vi "DiffIO Write.vi"(8 "FIFO Indexes.Write":cluster{"Diff I/O Setup":T1[]}, 9 "Command Enabled":bool, 11 "Device Inputs":dbl[](array[numeric])) -> (3 "Diff IO Setup":T2[](array[typedef]) {"Skip Fire Index" max=7; "Angles"."Duration [s]" format="%#_3p"; "Frequency [Hz]" format="%#_3p"})   [LabVIEW 2016, in "DCM Engine.lvlib"]
uses:
  DCM Engine.lvlib
  Built/DCM Classes Packed/Pharlap/C/DCM-Classes.lvlibp/DCM/Diff IO/RT/Setup.ctl
  Built/DCM Classes Packed/Pharlap/C/DCM-Classes.lvlibp/1abvi3w/vi.lib/Powertrain Controls/Device Drivers/DCM/Diff IO/FPGA/Mode.ctl
  Built/DCM Classes Packed/Pharlap/C/DCM-Classes.lvlibp/DCM/Diff IO/RT/Angle Control.ctl
  Shared/Types/DiffIO Setup Indexes.ctl
  Built/DCM Classes Packed/Pharlap/C/DCM-Classes.lvlibp/1abvi3w/vi.lib/Powertrain Controls/Device Drivers/DCM/Diff IO/FPGA/DCM - FPGA - Diff IO.lvlib
  Built/DCM Classes Packed/Pharlap/C/DCM-Classes.lvlibp/DCM/Diff IO/RT/DCM - RT - Diff IO.lvlib
  DCM Shared.lvlib
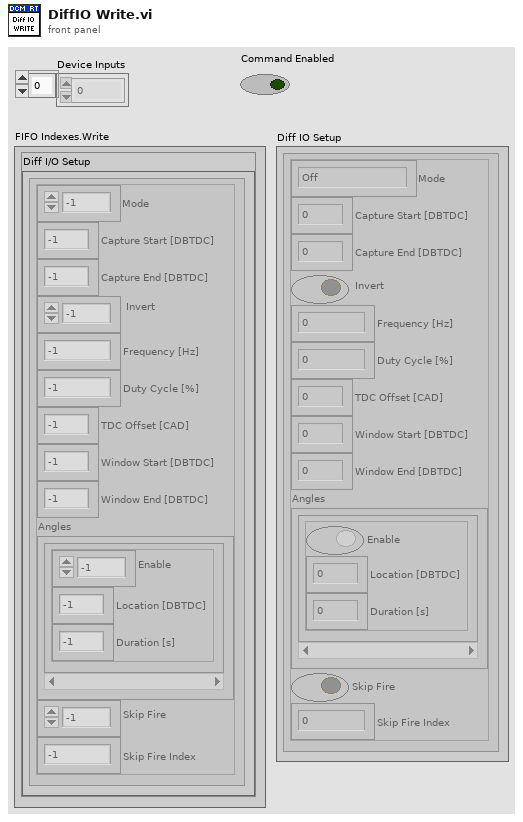
[diagram p1: front panel]
types:
  T1 = typedef "DCM Shared.lvlib/DiffIO Setup Indexes.ctl" = cluster{"Mode":i32, "Capture Start [DBTDC]":i32, "Capture End [DBTDC]":i32, "Invert":i32, "Frequency [Hz]":i32, "Duty Cycle [%]":i32, "TDC Offset [CAD]":i32, "Window Start [DBTDC]":i32, "Window End [DBTDC]":i32, "Angles":cluster{"Enable":i32, "Location [DBTDC]":i32, "Duration [s]":i32}[], "Skip Fire":i32, "Skip Fire Index":i32}
  T2 = typedef "DCM-Classes.lvlibp/DCM - RT - Diff IO.lvlib/Setup.ctl" = cluster{"Mode":T3, "Capture Start [DBTDC]":sgl, "Capture End [DBTDC]":sgl, "Invert":bool, "Frequency [Hz]":sgl, "Duty Cycle [%]":sgl, "TDC Offset [CAD]":sgl, "Window Start [DBTDC]":sgl, "Window End [DBTDC]":sgl, "Angles":T4[], "Skip Fire":bool, "Skip Fire Index":u8}
  T3 = typedef "DCM-Classes.lvlibp/DCM - FPGA - Diff IO.lvlib/Mode.ctl" = enum8{"Off", "Input", "Pulse Width Modulation", "Engine Position Tracking", "Serial Out 1", "Serial Out 2", "EPTx Sync"}
  T4 = typedef "DCM-Classes.lvlibp/DCM - RT - Diff IO.lvlib/Angle Control.ctl" = cluster{"Enable":bool, "Location [DBTDC]":sgl, "Duration [s]":sgl}
  T5 = cluster{"Enable":i32, "Location [DBTDC]":i32, "Duration [s]":i32}[]
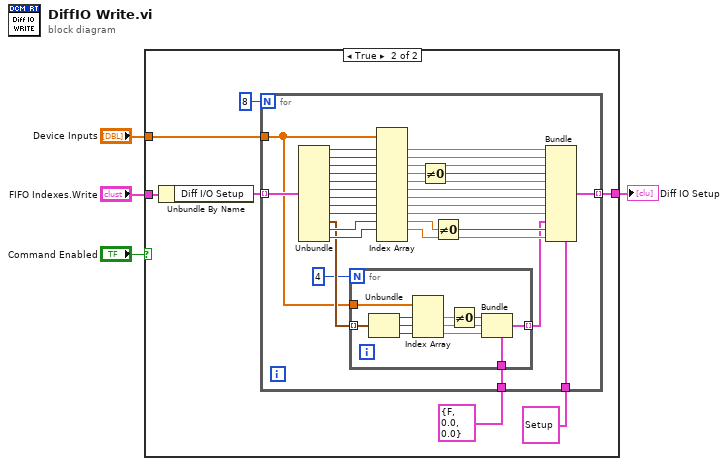
[diagram p0: block diagram]
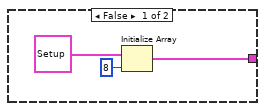
[diagram p2: hidden frame]
diagram:
  n1 = case shown="True" "Command Enabled" {
    tunnel: "Device Inputs" -> [_ w14]
    tunnel: [w5 w12] -> w3
    tunnel: "FIFO Indexes.Write" -> [_ w9]
    frame False {
      n2 = Initialize Array(T2 {"Mode"=enum."Off", "Capture Start [DBTDC]"=0.0, "Capture End [DBTDC]"=0.0, "Invert"=FALSE, "Frequency [Hz]"=0.0, "Duty Cycle [%]"=0.0, "TDC Offset [CAD]"=0.0, "Window Start [DBTDC]"=0.0, "Window End [DBTDC]"=0.0, "Angles"=[{"Enable"=FALSE, "Location [DBTDC]"=0.0, "Duration [s]"=0.0}, {"Enable"=FALSE, "Location [DBTDC]"=0.0, "Duration [s]"=0.0}, {"Enable"=FALSE, "Location [DBTDC]"=0.0, "Duration [s]"=0.0}, {"Enable"=FALSE, "Location [DBTDC]"=0.0, "Duration [s]"=0.0}], "Skip Fire"=FALSE, "Skip Fire Index"=0} ("PWM Control 2"), 8 ("dimension size")) -> (w5:T2[])
    }
    frame True {
      n3 = Unbundle By Name(w9) -> ("Diff I/O Setup"=w13:T1[])
      n4 = for {
        N: 8 -> [_]
        tunnel: w14 -> [w33]
        tunnel: w13 -> [w46] mode=indexing
        tunnel: [w32] -> w12 mode=indexing
        tunnel: T4 {"Enable"=FALSE, "Location [DBTDC]"=0.0, "Duration [s]"=0.0} ("Injection Control") -> [w31]
        tunnel: T2 {"Mode"=enum."Off", "Capture Start [DBTDC]"=0.0, "Capture End [DBTDC]"=0.0, "Invert"=FALSE, "Frequency [Hz]"=0.0, "Duty Cycle [%]"=0.0, "TDC Offset [CAD]"=0.0, "Window Start [DBTDC]"=0.0, "Window End [DBTDC]"=0.0, "Angles"=[{"Enable"=FALSE, "Location [DBTDC]"=0.0, "Duration [s]"=0.0}, {"Enable"=FALSE, "Location [DBTDC]"=0.0, "Duration [s]"=0.0}, {"Enable"=FALSE, "Location [DBTDC]"=0.0, "Duration [s]"=0.0}, {"Enable"=FALSE, "Location [DBTDC]"=0.0, "Duration [s]"=0.0}], "Skip Fire"=FALSE, "Skip Fire Index"=0} ("PWM Control 2") -> [w15]
        n5 = Unbundle(w46) -> ("Mode"=w45:i32, "Capture Start [DBTDC]"=w44:i32, "Capture End [DBTDC]"=w43:i32, "Invert"=w42:i32, "Frequency [Hz]"=w41:i32, "Duty Cycle [%]"=w40:i32, "TDC Offset [CAD]"=w39:i32, "Window Start [DBTDC]"=w38:i32, "Window End [DBTDC]"=w37:i32, "Angles"=w34:T5, "Skip Fire"=w36:i32, "Skip Fire Index"=w35:i32)
        n6 = for {
          N: 4 -> [_]
          tunnel: w34 -> [w56] mode=indexing
          tunnel: w33 -> [w57]
          tunnel: w31 -> [w52]
          tunnel: [w47] -> w18 mode=indexing
          n7 = Unbundle(w56) -> ("Enable"=w55:i32, "Location [DBTDC]"=w54:i32, "Duration [s]"=w53:i32)
          n8 = Index Array(array=w57, index #1=w55, index #2=w54, index #3=w53) -> (element #1=w51:dbl, element #2=w49:dbl, element #3=w48:dbl)
          n9 = Not Equal To 0?(x=w51) -> (x != 0?=w50:bool)
          n10 = Bundle(cluster=w52, "Enable"=w50, "Location [DBTDC]"=w49, "Duration [s]"=w48) -> (w47:T4)
        }
        n11 = Index Array(array=w33, index #1=w45, index #2=w44, index #3=w43, index #4=w42, index #5=w41, index #6=w40, index #7=w39, index #8=w38, index #9=w37, index #10=w36, index #11=w35) -> (element #1=w17:dbl, element #2=w30:dbl, element #3=w29:dbl, element #4=w22:dbl, element #5=w28:dbl, element #6=w27:dbl, element #7=w26:dbl, element #8=w25:dbl, element #9=w24:dbl, element #10=w20:dbl, element #11=w23:dbl)  [unwired: 1 in, 1 out]
        n12 = Not Equal To 0?(x=w22) -> (x != 0?=w21:bool)
        n13 = Not Equal To 0?(x=w20) -> (x != 0?=w19:bool)
        n14 = Bundle(cluster=w15, "Mode"=w17, "Capture Start [DBTDC]"=w30, "Capture End [DBTDC]"=w29, "Invert"=w21, "Frequency [Hz]"=w28, "Duty Cycle [%]"=w27, "TDC Offset [CAD]"=w26, "Window Start [DBTDC]"=w25, "Window End [DBTDC]"=w24, "Angles"=w18, "Skip Fire"=w19, "Skip Fire Index"=w23) -> (w32:T2)
      }
    }
  }
  "Diff IO Setup" <- w3
